vi "find_first_photon.vi"(11 "timetags":u32[][](array[numeric])) -> (3 "Numeric":dbl)   [LabVIEW 2018]
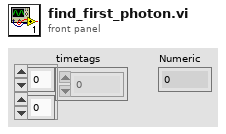
[diagram p1: front panel]
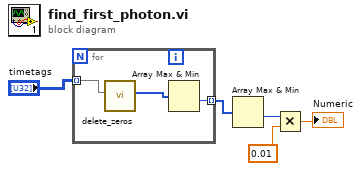
[diagram p0: block diagram]
diagram:
  n1 = for {
    tunnel: "timetags" -> [w8] mode=indexing
    tunnel: [w6] -> w3 mode=indexing
    n2 = call "delete_zeros.vi"("array_in"=w8) -> ("array_out"=w7:u32[])  [unwired: 10 in]
    n3 = Array Max & Min(array=w7) -> (min value=w6:u32)  [unwired: 3 out]
  }
  n4 = Array Max & Min(array=w3) -> (min value=w4:u32)  [unwired: 3 out]
  n5 = Multiply(x=w4, y=0.01) -> (x*y=→"Numeric":dbl)
